vi "S-ParmsSetup.vi"(0 "VISA IN":refnum<visa-resource-name>, 5 "error in":errorcluster) -> (14 "VISA Out":refnum<visa-resource-name>, 19 "error out":errorcluster)   [LabVIEW 2018, in "PNA-X.lvlib"]
uses:
  PNA-X.lvlib
panel:
  in  "Window Function":i32(slide) min=0 max=2 step=1 scale=0.0..2.0
  out "Data":string
  in  "Measurement Parameter in Quotes":string
  in  "Measurement Name in Quotes":string
  in  "Trace":i32=1
  in  "Window":i32=1
  in  "Channel":i32=1
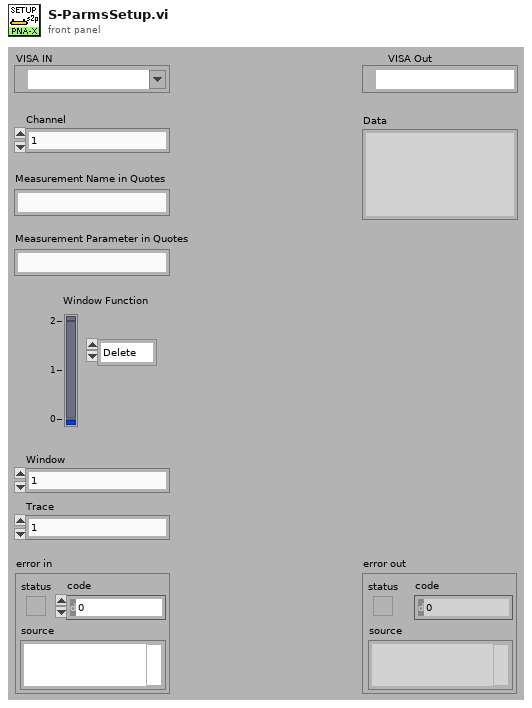
[diagram p1: front panel]
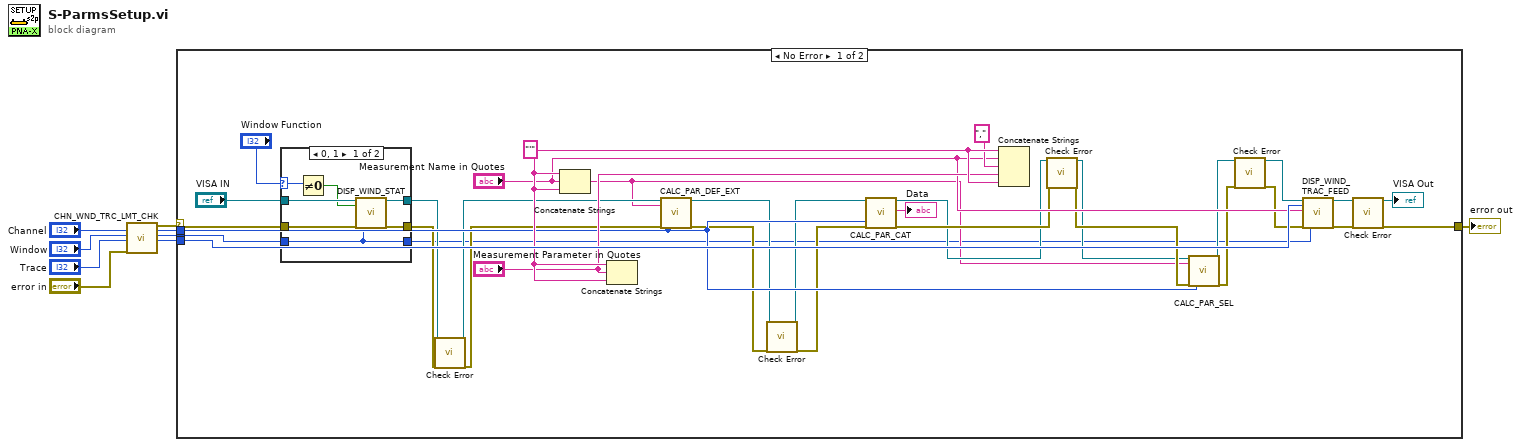
[diagram p0: block diagram]
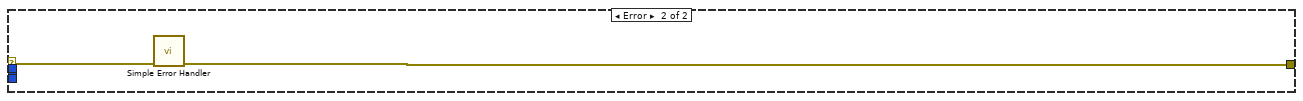
[diagram p3: hidden frame]
diagram:
  n1 = call "CHN_WND_TRC_LMT_CHK.vi"("Channel"="Channel", "Window"="Window", "Trace"="Trace", "error in"="error in") -> ("error out"=w4:errorcluster, "Channel"=w1:i32, "Window"=w3:i32, "Trace"=w2:i32)  [unwired: 11 in, 1 out]
  n2 = case shown="No Error" w4 {
    selector: w4 -> [w37 w54]
    tunnel: [w42 w53] -> w6
    tunnel: w3 -> [w10 _]
    tunnel: w2 -> [w36 _]
    tunnel: w1 -> [w31 _]
    frame No Error {
      w35 = "'"
      n3 = case shown="0, 1" "Window Function" {
        selector: "Window Function" -> [w44 _]
        tunnel: "VISA IN" -> [w49 w51]
        tunnel: w37 -> [w48 w52]
        tunnel: w10 -> [w45 w50]
        tunnel: [w47 w51] -> w17
        tunnel: [w46 w52] -> w15
        tunnel: [w45 w50] -> w12
        frame 0, 1 {
          n4 = Not Equal To 0?(x=w44) -> (x != 0?=w43:bool)
          n5 = call "DISP_WIND_STAT.vi"("VISA IN"=w49, "ON | OFF"=w43, "error in"=w48, "Window"=w45) -> ("VISA Out"=w47:refnum<visa-resource-name>, "error out"=w46:errorcluster)  [unwired: 14 in]
        }
        frame 2, Default {
        }
      }
      n6 = call "Check Error.vi"("VISA Resource Name"=w17, "error in (no error)"=w15) -> ("dup VISA session"=w16:refnum<visa-resource-name>, "error out"=w14:errorcluster)  [unwired: 16 in]
      n7 = Concatenate Strings(w35, "Measurement Name in Quotes", w35) -> (w13:string)
      n8 = Concatenate Strings(w35, "Measurement Parameter in Quotes", w35) -> ()  [unwired: 1 out]
      n9 = call "CALC_PAR_DEF_EXT.vi"("VISA IN"=w16, "Measurement Name"=w13, "error in"=w14, "Channel"=w31) -> ("VISA Out"=w21:refnum<visa-resource-name>, "error out"=w20:errorcluster)  [unwired: 12 in, 2 out]
      n10 = call "Check Error.vi"("VISA Resource Name"=w21, "error in (no error)"=w20) -> ("dup VISA session"=w18:refnum<visa-resource-name>, "error out"=w19:errorcluster)  [unwired: 16 in]
      n11 = call "CALC_PAR_CAT.vi"("VISA IN"=w18, "error in"=w19, "Channel"=w31) -> ("VISA Out"=w24:refnum<visa-resource-name>, "Data"=→"Data":string, "error out"=w25:errorcluster)  [unwired: 12 in, 2 out]
      n12 = Concatenate Strings(w35, "Measurement Name in Quotes", ",", "Measurement Parameter in Quotes", w35) -> ()  [unwired: 1 out]
      n13 = call "Check Error.vi"("VISA Resource Name"=w24, "error in (no error)"=w25) -> ("dup VISA session"=w22:refnum<visa-resource-name>, "error out"=w23:errorcluster)  [unwired: 16 in]
      n14 = call "CALC_PAR_SEL.vi"("VISA IN"=w22, "Measurement"=w13, "error in"=w23, "Channel"=w31) -> ("VISA Out"=w29:refnum<visa-resource-name>, "error out"=w28:errorcluster)  [unwired: 14 in]
      n15 = call "Check Error.vi"("VISA Resource Name"=w29, "error in (no error)"=w28) -> ("dup VISA session"=w27:refnum<visa-resource-name>, "error out"=w26:errorcluster)  [unwired: 16 in]
      n16 = call "DISP_WIND_TRAC_FEED.vi"("VISA IN"=w27, "Trace"=w36, "Name"="Measurement Name in Quotes", "error in"=w26, "Window"=w12) -> ("VISA Out"=w39:refnum<visa-resource-name>, "error out"=w38:errorcluster)  [unwired: 13 in]
      n17 = call "Check Error.vi"("VISA Resource Name"=w39, "error in (no error)"=w38) -> ("dup VISA session"=→"VISA Out":refnum<visa-resource-name>, "error out"=w42:errorcluster)  [unwired: 16 in]
    }
    frame Error {
      n18 = call <vilib>:"Simple Error Handler.vi"("error in (no error)"=w54) -> ("error out"=w53:errorcluster)  [unwired: 4 in, 4 out]
    }
  }
  "error out" <- w6
